vi "DIO_OFF.vi"(8 "error in (no error)":errorcluster, 11 "IN":T1={"step name 1"="", "updata 2"="1000", "limitdata 3"="", "load vi name 4"="", "parameter 5"="port0~line0"}) -> (0 "error out":errorcluster, 3 "Cluster":T2)   [LabVIEW 2013]
uses:
  SubVi/Global constant.vi
panel:
  out "concatenated string":string
  # "port0~line0"
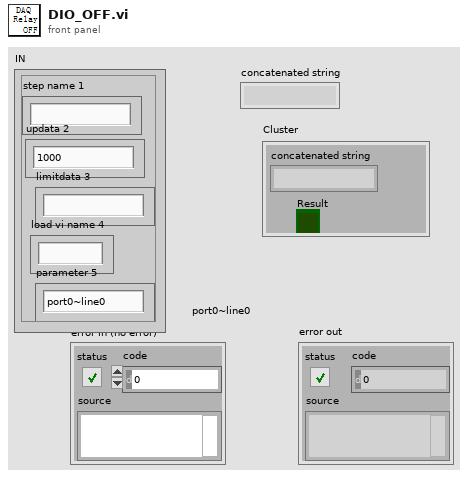
[diagram p1: front panel]
types:
  T1 = cluster{"step name 1":string, "updata 2":string, "limitdata 3":string, "load vi name 4":string, "parameter 5":string}
  T2 = cluster{"concatenated string":string, "Result":bool}
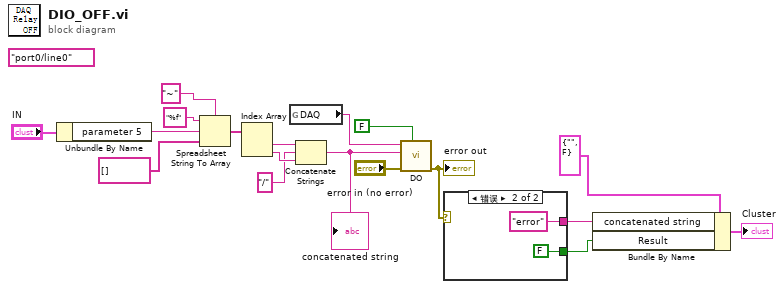
[diagram p0: block diagram]
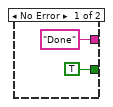
[diagram p2: hidden frame]
diagram:
  (unwired) "port0/line0" ("Line")
  n1 = Unbundle By Name("IN") -> ("parameter 5"=w8:string)
  n2 = Spreadsheet String To Array(delimiter (Tab)="~", format string="%f", spreadsheet string=w8, array type (2D Dbl)=string[] []) -> (array=w5:string[])
  n3 = Index Array(array=w5) -> (element #1=w4:string, element #2=w3:string)  [unwired: 2 in]
  n4 = global read "Global constant.vi" "DAQ"() -> (w14:tag)
  n5 = Concatenate Strings(w4, "/" ("string"), w3) -> (w1:string)
  "concatenated string" <- w1
  n6 = call "DO.vi"("ON?"=FALSE, "error in"="error in (no error)", "Line"=w1, "Device"=w14) -> ("error out"=w13:errorcluster)  [unwired: 7 in]
  "error out" <- w13
  n7 = case shown="错误" w13 {
    tunnel: [TRUE FALSE] -> w12
    tunnel: ["Done" "error"] -> w11
    frame No Error {
    }
    frame Error {
    }
  }
  n8 = Bundle By Name(cluster=T2 {"concatenated string"="", "Result"=FALSE} ("Cluster"), "concatenated string"=w11, "Result"=w12) -> (→"Cluster":T2)
